vi "get_config_path.vi"(6 "configuration":T1, 8 "error in (no error)":errorcluster, 11 "custom_file":path) -> (0 "error out":errorcluster, 3 "config_path":path)   [LabVIEW 2015, in "lv-builder-l3.lvlib"]
uses:
  lv-builder-l3.lvlib
  public/_controls/configuration.ctl
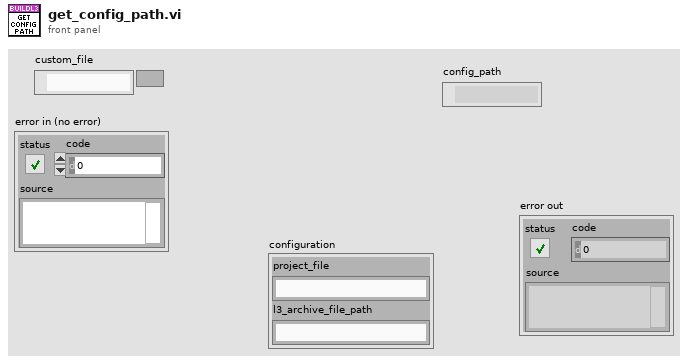
[diagram p1: front panel]
types:
  T1 = typedef "lv-builder-l3.lvlib/configuration.ctl" = cluster{"project_file":string, "l3_archive_file_path":string}
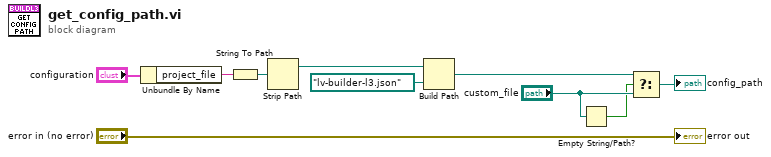
[diagram p0: block diagram]
diagram:
  n1 = Unbundle By Name("configuration") -> ("project_file"=w7:string)
  n2 = String To Path(string=w7) -> (path=w6:path)
  n3 = Strip Path(path=w6) -> (stripped path=w9:path)  [unwired: 1 out]
  n4 = Build Path(base path=w9, name or relative path=path "lv-builder-l3.json" ("stripped path")) -> (appended path=w5:path)
  n5 = Empty String/Path?(string/path="custom_file") -> (empty?=w2:bool)
  n6 = Select(t=w5, s=w2, f="custom_file") -> (s? t:f=→"config_path":path)
  "error out" <- "error in (no error)"
